vi "Parse Numeric.vi"(8 "error in (no error)":errorcluster, 10 "Index In":i32, 11 "JSON String":string) -> (0 "error out":errorcluster, 2 "Index Out":i32, 3 "JSON Numeric out":refnum<class "JSON Numeric.lvclass">)   [LabVIEW 2016, in "LVJSON.lvlib" / "JSON Helper.lvclass"]
uses:
  JSON Helper.lvclass
  JSON Numeric/JSON Numeric.lvclass
  Errors/Errors.ctl
  JSON Numeric/New JSON Numeric.vi
  LVJSON.lvlib
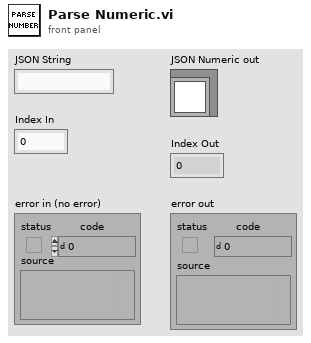
[diagram p1: front panel]
types:
  T1 = typedef "LVJSON.lvlib/Errors.ctl" = enum16{"No key", "Key path type", "Array OOB", "Type Mismatch", "Invalid Token"}
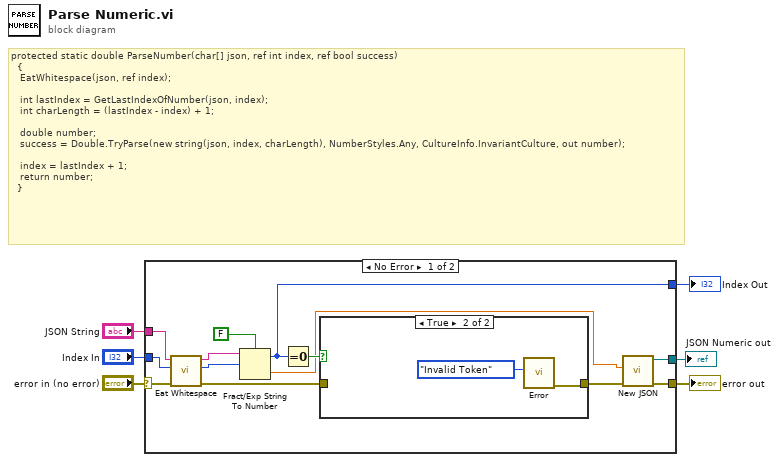
[diagram p0: block diagram]
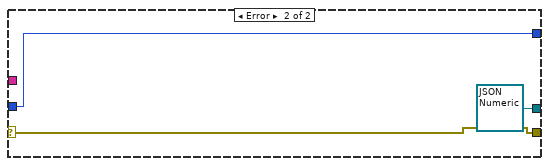
[diagram p3: hidden frame]
diagram:
  # "protected static double ParseNumber(char[] json, ref int index, ref bool success)\n\t\t{\n\t\t\tEatWhitespace(json, ref index);\n\n\t\t\tint lastIndex = GetLastIndexOfNumber(json, index);\n\t\t\tint charLength = (lastIndex - index) + 1;\n\n\t\t\tdouble number;\n\t\t\tsuccess = Double.TryParse(new string(json, index, charLength), NumberStyles.Any, CultureInfo.InvariantCulture, out number);\n\n\t\t\tindex = lastIndex + 1;\n\t\t\treturn number;\n\t\t}"
  n1 = case shown="No Error" "error in (no error)" {
    selector: "error in (no error)" -> [w18 w24]
    tunnel: [w14 w24] -> w5
    tunnel: [w13 refnum<class "JSON Numeric.lvclass"> refnum ("JSON String out")] -> w1
    tunnel: "Index In" -> [w19 w25]
    tunnel: [w15 w25] -> w3
    tunnel: "JSON String" -> [w8 _]
    frame No Error {
      n2 = call "Eat Whitespace.vi"("error in (no error)"=w18, "Index In"=w19, "JSON String"=w8) -> ("error out"=w11:errorcluster, "Index Out"=w16:i32, "JSON String Passthrough"=w17:string)  [unwired: 6 in]
      n3 = Fract/Exp String To Number(use system decimal point (T)=FALSE, string=w17, offset=w16) -> (offset past number=w15:i32, number=w7:dbl)  [unwired: 1 in]
      n4 = Equal To 0?(x=w15) -> (x = 0?=w12:bool)
      n5 = case shown="True" w12 {
        tunnel: w11 -> [w20 _]
        tunnel: [w20 w22] -> w10
        frame False {
        }
        frame True {
          n6 = call "Error.vi"(9:Errors."Invalid Token") -> ("error out"=w22:errorcluster)  [unwired: 9 in]
        }
      }
      n7 = call-poly "New JSON.vi"("error in (no error)"=w10, "value"=w7) -> ("error out"=w14:errorcluster, "JSON String out"=w13:refnum<class "JSON Numeric.lvclass">)  [unwired: 8 in]
    }
    frame Error {
    }
  }
  "error out" <- w5
  "Index Out" <- w3
  "JSON Numeric out" <- w1
